vi "SetSubPanelRef.vi"(8 "error in (no error)":errorcluster, 10 "SubPanelReference":refnum<vi>, 11 "EmbeddedSMO in":refnum<class "Embedded UI.lvclass">) -> (0 "error out":errorcluster, 3 "EmbeddedSMO out":refnum<class "Embedded UI.lvclass">)   [LabVIEW 2019, in "Embedded UI.lvclass"]
uses:
  Embedded UI.lvclass
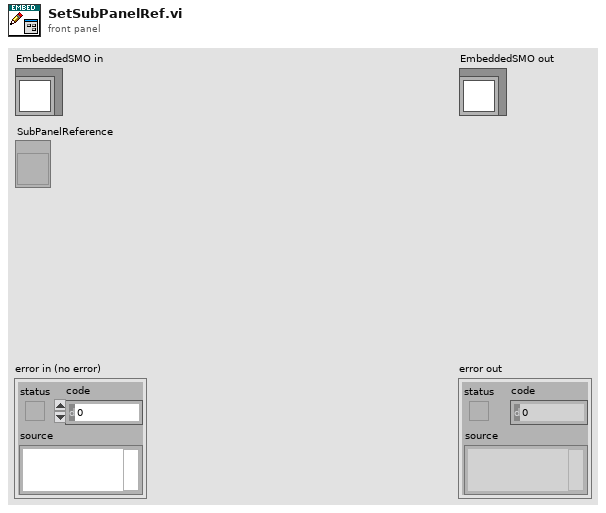
[diagram p1: front panel]
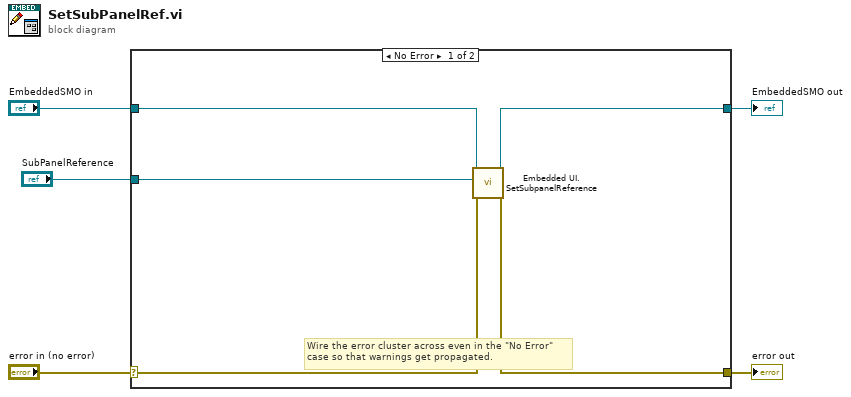
[diagram p0: block diagram]
diagram:
  n1 = case shown="No Error" "error in (no error)" {
    selector: "error in (no error)" -> [w9 w12]
    tunnel: [w8 w12] -> w4
    tunnel: [w10 w11] -> w2
    tunnel: "EmbeddedSMO in" -> [w7 w11]
    tunnel: "SubPanelReference" -> [w6 _]
    frame No Error {
      # "Wire the error cluster across even in the \"No Error\"\ncase so that warnings get propagated."
      n2 = call "Embedded UI.SetSubpanelReference.vi"("error in (no error)"=w9, "SetSubpanelReference"=w6, "EmbeddedSMO"=w7) -> ("error out"=w8:errorcluster, "EmbeddedSMO out"=w10:refnum<class "Embedded UI.lvclass">)  [unwired: 7 in]
    }
    frame Error {
    }
  }
  "error out" <- w4
  "EmbeddedSMO out" <- w2
